vi "PID Calculate Gains.vi"(3 "PID parameters":cluster{"Kc":dbl, "Ti":dbl, "Td":dbl} {"Td" format="%.2f"; "Ti" format="%.2f"; "Kc" format="%.2f"}, 4 "autotuning parameters":T1={"Controller Type"=0, "# of cycles to avg"=3, "Relay amplitude (%)"=0.0, "Control design  "=0, "Noise level %"=0.25} {"Noise level %" format="%.2f"; "Control design" items=["Normal", "Fast", "Slow"]; "Relay amplitude (%)" format="%.2f"; "Controller Type" items=["PID", "PI", "P"]}, 5 "Mean amplitude":dbl format="%.2f", 6 "Mean period":dbl format="%.2f") -> (0 "tuned PID parameters":cluster{"Kc":dbl, "Ti":dbl, "Td":dbl} {"Td" format="%.2f"; "Ti" format="%.2f"; "Kc" format="%.2f"}, 1 "Tu":dbl format="%.2f", 2 "Kr":dbl)   [LabVIEW 2020, in "NI_PID_autopid.lvlib"]
doc: "This VI determines the new PID parameters from the results of the setpoint relay experiment."
uses:
  <vilib>/addons/control/pid/NI_PID_autopid.lvlib
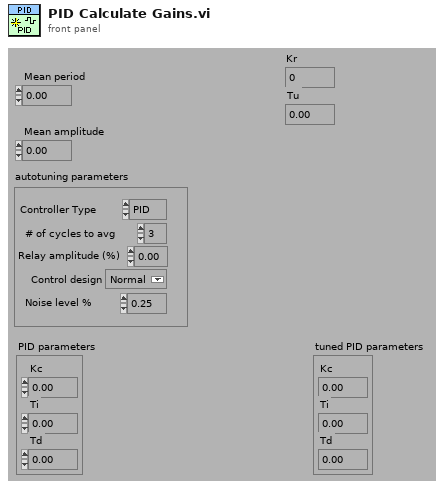
[diagram p1: front panel]
types:
  T1 = cluster{"Controller Type":u16, "# of cycles to avg":i32, "Relay amplitude (%)":dbl, "Control design  ":u16, "Noise level %":dbl}
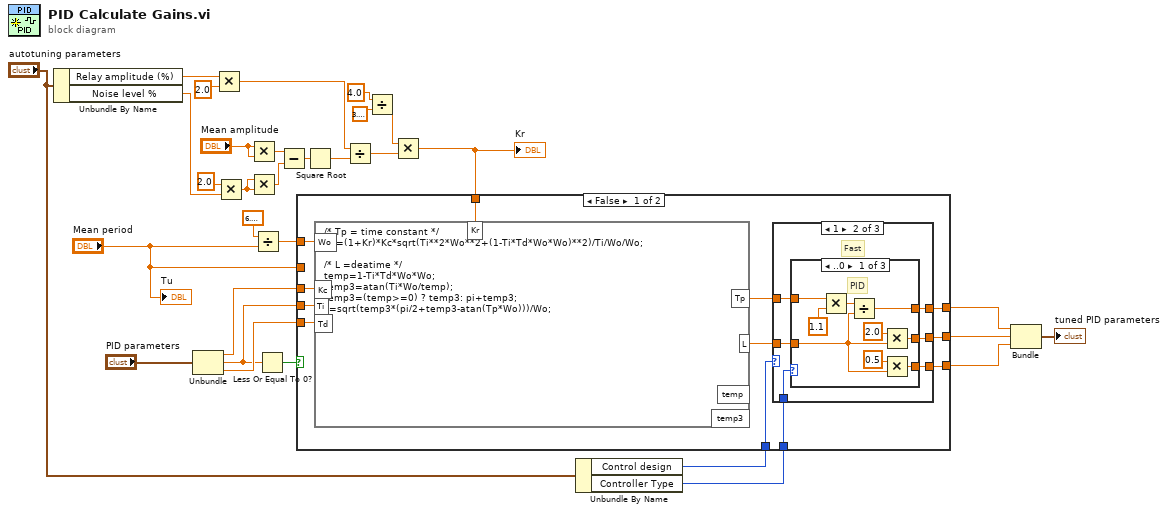
[diagram p0: block diagram]
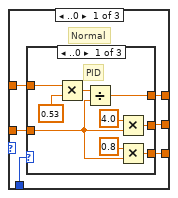
[diagram p2: hidden frame]
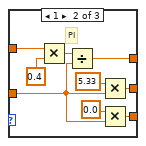
[diagram p3: hidden frame]
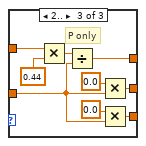
[diagram p4: hidden frame]
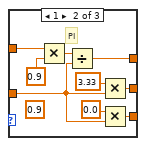
[diagram p5: hidden frame]
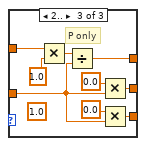
[diagram p6: hidden frame]
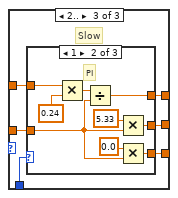
[diagram p7: hidden frame]
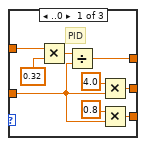
[diagram p8: hidden frame]
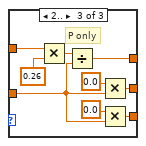
[diagram p9: hidden frame]
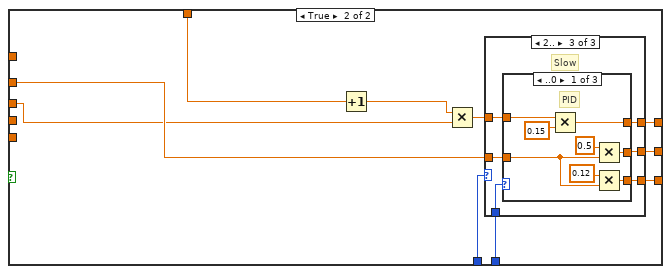
[diagram p10: hidden frame]
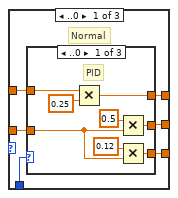
[diagram p11: hidden frame]
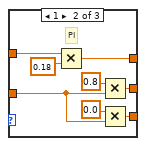
[diagram p12: hidden frame]
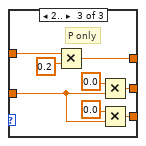
[diagram p13: hidden frame]
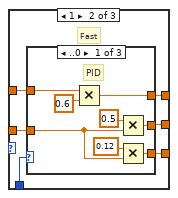
[diagram p14: hidden frame]
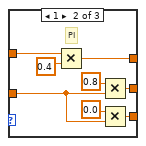
[diagram p15: hidden frame]
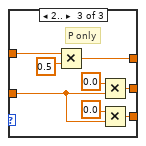
[diagram p16: hidden frame]
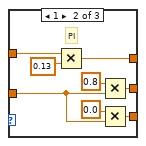
[diagram p17: hidden frame]
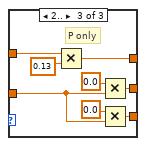
[diagram p18: hidden frame]
diagram:
  n1 = Unbundle By Name("autotuning parameters") -> ("Relay amplitude (%)"=w15:dbl, "Noise level %"=w1:dbl)
  n2 = Unbundle("PID parameters") -> ("Kc"=w5:dbl, "Ti"=w19:dbl, "Td"=w20:dbl)
  n3 = Multiply(x=w15, y=2.0) -> (x*y=w29:dbl)
  n4 = Multiply(x=2.0, y=w1) -> (x*y=w24:dbl)
  n5 = Multiply(x="Mean amplitude", y="Mean amplitude") -> (x*y=w26:dbl)
  n6 = Multiply(x=w24, y=w24) -> (x*y=w22:dbl)
  n7 = Divide(x=6.283185307179586, y="Mean period") -> (x/y=w8:dbl)
  n8 = Less Or Equal To 0?(x=w19) -> (x <= 0?=w30:bool)
  n9 = Subtract(x=w26, y=w22) -> (x-y=w23:dbl)
  n10 = Square Root(x=w23) -> (sqrt(x)=w25:dbl)
  n11 = Divide(x=w29, y=w25) -> (x/y=w27:dbl)
  n12 = Divide(x=4.0, y=3.141592653589793) -> (x/y=w11:dbl)
  n13 = Multiply(x=w11, y=w27) -> (x*y=w28:dbl)
  "Kr" <- w28
  n14 = Unbundle By Name("autotuning parameters") -> ("Control design"=w10:u16, "Controller Type"=w9:u16)
  n15 = case shown="False" w30 {
    tunnel: w20 -> [w43 _]
    tunnel: w19 -> [w42 _]
    tunnel: w28 -> [w41 w148]
    tunnel: [w34 w146] -> w4
    tunnel: [w33 w145] -> w21
    tunnel: w5 -> [w40 w143]
    tunnel: w10 -> [w37 w152]
    tunnel: w9 -> [w36 w151]
    tunnel: w8 -> [w35 _]
    tunnel: "Mean period" -> [_ w150]
    tunnel: [w32 w144] -> w6
    frame False {
      n16 = formula code="/* Tp = time constant */\nTp=(1+Kr)*Kc*sqrt(Ti**2*Wo**2+(1-Ti*Td*Wo*Wo)**2)/Ti/Wo/Wo;\n\n/* L =deatime */\ntemp=1-Ti*Td*Wo*Wo;\ntemp3=atan(Ti*Wo/temp);\ntemp3=(temp>=0) ? temp3: pi+temp3;\nL=sqrt(temp3*(pi/2+temp3-atan(Tp*Wo)))/Wo;"("Wo"=w35, "Kr"=w41, "Ti"=w42, "Td"=w43, "Kc"=w40) -> ("Tp"=w38:dbl, "L"=w39:dbl)  [unwired: 2 out]
      n17 = case shown="1" w37 {
        tunnel: [w49 w78 w113] -> w33
        tunnel: [w48 w79 w114] -> w32
        tunnel: [w47 w80 w115] -> w34
        tunnel: w39 -> [w46 w81 w112]
        tunnel: w38 -> [w45 w82 w111]
        tunnel: w36 -> [w44 w77 w110]
        frame ..0 {
          # "Normal"
          n18 = case shown="..0" w44 {
            tunnel: [w50 w59 w68] -> w47
            tunnel: [w55 w64 w73] -> w49
            tunnel: w46 -> [w54 w63 w72]
            tunnel: [w51 w60 w69] -> w48
            tunnel: w45 -> [w52 w61 w70]
            frame ..0 {
              # "PID"
              n19 = Multiply(x=w52, y=0.53) -> (x*y=w58:dbl)
              n20 = Divide(x=w58, y=w54) -> (x/y=w50:dbl)
              n21 = Multiply(x=4.0, y=w54) -> (x*y=w51:dbl)
              n22 = Multiply(x=0.8, y=w54) -> (x*y=w55:dbl)
            }
            frame 1 {
              # "PI"
              n23 = Multiply(x=w61, y=0.4) -> (x*y=w67:dbl)
              n24 = Divide(x=w67, y=w63) -> (x/y=w59:dbl)
              n25 = Multiply(x=5.33, y=w63) -> (x*y=w60:dbl)
              n26 = Multiply(x=0.0, y=w63) -> (x*y=w64:dbl)
            }
            frame 2.. {
              # "P only"
              n27 = Multiply(x=w70, y=0.44) -> (x*y=w76:dbl)
              n28 = Divide(x=w76, y=w72) -> (x/y=w68:dbl)
              n29 = Multiply(x=0.0, y=w72) -> (x*y=w69:dbl)
              n30 = Multiply(x=0.0, y=w72) -> (x*y=w73:dbl)
            }
          }
        }
        frame 1 {
          # "Fast"
          n31 = case shown="..0" w77 {
            tunnel: [w83 w92 w101] -> w80
            tunnel: [w88 w97 w106] -> w78
            tunnel: w81 -> [w87 w96 w105]
            tunnel: [w84 w93 w102] -> w79
            tunnel: w82 -> [w85 w94 w103]
            frame ..0 {
              # "PID"
              n32 = Multiply(x=w85, y=1.1) -> (x*y=w91:dbl)
              n33 = Divide(x=w91, y=w87) -> (x/y=w83:dbl)
              n34 = Multiply(x=2.0, y=w87) -> (x*y=w84:dbl)
              n35 = Multiply(x=0.5, y=w87) -> (x*y=w88:dbl)
            }
            frame 1 {
              (unwired) 0.9
              # "PI"
              n36 = Multiply(x=w94, y=0.9) -> (x*y=w100:dbl)
              n37 = Divide(x=w100, y=w96) -> (x/y=w92:dbl)
              n38 = Multiply(x=3.33, y=w96) -> (x*y=w93:dbl)
              n39 = Multiply(x=0.0, y=w96) -> (x*y=w97:dbl)
            }
            frame 2.. {
              (unwired) 1.0
              # "P only"
              n40 = Multiply(x=w103, y=1.0) -> (x*y=w109:dbl)
              n41 = Divide(x=w109, y=w105) -> (x/y=w101:dbl)
              n42 = Multiply(x=0.0, y=w105) -> (x*y=w102:dbl)
              n43 = Multiply(x=0.0, y=w105) -> (x*y=w106:dbl)
            }
          }
        }
        frame 2.. {
          # "Slow"
          n44 = case shown="1" w110 {
            tunnel: [w116 w125 w134] -> w115
            tunnel: [w121 w130 w139] -> w113
            tunnel: w112 -> [w120 w129 w138]
            tunnel: [w117 w126 w135] -> w114
            tunnel: w111 -> [w118 w127 w136]
            frame ..0 {
              # "PID"
              n45 = Multiply(x=w118, y=0.32) -> (x*y=w124:dbl)
              n46 = Divide(x=w124, y=w120) -> (x/y=w116:dbl)
              n47 = Multiply(x=4.0, y=w120) -> (x*y=w117:dbl)
              n48 = Multiply(x=0.8, y=w120) -> (x*y=w121:dbl)
            }
            frame 1 {
              # "PI"
              n49 = Multiply(x=w127, y=0.24) -> (x*y=w133:dbl)
              n50 = Divide(x=w133, y=w129) -> (x/y=w125:dbl)
              n51 = Multiply(x=5.33, y=w129) -> (x*y=w126:dbl)
              n52 = Multiply(x=0.0, y=w129) -> (x*y=w130:dbl)
            }
            frame 2.. {
              # "P only"
              n53 = Multiply(x=w136, y=0.26) -> (x*y=w142:dbl)
              n54 = Divide(x=w142, y=w138) -> (x/y=w134:dbl)
              n55 = Multiply(x=0.0, y=w138) -> (x*y=w135:dbl)
              n56 = Multiply(x=0.0, y=w138) -> (x*y=w139:dbl)
            }
          }
        }
      }
    }
    frame True {
      n57 = Increment(x=w148) -> (x+1=w147:dbl)
      n58 = Multiply(x=w147, y=w143) -> (x*y=w149:dbl)
      n59 = case shown="2.." w152 {
        tunnel: [w158 w188 w218] -> w145
        tunnel: [w157 w187 w217] -> w144
        tunnel: [w156 w186 w216] -> w146
        tunnel: w150 -> [w155 w185 w215]
        tunnel: w149 -> [w154 w184 w214]
        tunnel: w151 -> [w153 w183 w213]
        frame ..0 {
          # "Normal"
          n60 = case shown="..0" w153 {
            tunnel: [w159 w167 w175] -> w156
            tunnel: [w164 w172 w180] -> w158
            tunnel: w155 -> [w163 w171 w179]
            tunnel: [w160 w168 w176] -> w157
            tunnel: w154 -> [w161 w169 w177]
            frame ..0 {
              # "PID"
              n61 = Multiply(x=w161, y=0.25) -> (x*y=w159:dbl)
              n62 = Multiply(x=0.5, y=w163) -> (x*y=w160:dbl)
              n63 = Multiply(x=0.12, y=w163) -> (x*y=w164:dbl)
            }
            frame 1 {
              # "PI"
              n64 = Multiply(x=w169, y=0.18) -> (x*y=w167:dbl)
              n65 = Multiply(x=0.8, y=w171) -> (x*y=w168:dbl)
              n66 = Multiply(x=0.0, y=w171) -> (x*y=w172:dbl)
            }
            frame 2.. {
              # "P only"
              n67 = Multiply(x=w177, y=0.2) -> (x*y=w175:dbl)
              n68 = Multiply(x=0.0, y=w179) -> (x*y=w176:dbl)
              n69 = Multiply(x=0.0, y=w179) -> (x*y=w180:dbl)
            }
          }
        }
        frame 1 {
          # "Fast"
          n70 = case shown="..0" w183 {
            tunnel: [w189 w197 w205] -> w186
            tunnel: [w194 w202 w210] -> w188
            tunnel: w185 -> [w193 w201 w209]
            tunnel: [w190 w198 w206] -> w187
            tunnel: w184 -> [w191 w199 w207]
            frame ..0 {
              # "PID"
              n71 = Multiply(x=w191, y=0.6) -> (x*y=w189:dbl)
              n72 = Multiply(x=0.5, y=w193) -> (x*y=w190:dbl)
              n73 = Multiply(x=0.12, y=w193) -> (x*y=w194:dbl)
            }
            frame 1 {
              # "PI"
              n74 = Multiply(x=w199, y=0.4) -> (x*y=w197:dbl)
              n75 = Multiply(x=0.8, y=w201) -> (x*y=w198:dbl)
              n76 = Multiply(x=0.0, y=w201) -> (x*y=w202:dbl)
            }
            frame 2.. {
              # "P only"
              n77 = Multiply(x=w207, y=0.5) -> (x*y=w205:dbl)
              n78 = Multiply(x=0.0, y=w209) -> (x*y=w206:dbl)
              n79 = Multiply(x=0.0, y=w209) -> (x*y=w210:dbl)
            }
          }
        }
        frame 2.. {
          # "Slow"
          n80 = case shown="..0" w213 {
            tunnel: [w219 w227 w235] -> w216
            tunnel: [w224 w232 w240] -> w218
            tunnel: w215 -> [w223 w231 w239]
            tunnel: [w220 w228 w236] -> w217
            tunnel: w214 -> [w221 w229 w237]
            frame ..0 {
              # "PID"
              n81 = Multiply(x=w221, y=0.15) -> (x*y=w219:dbl)
              n82 = Multiply(x=0.5, y=w223) -> (x*y=w220:dbl)
              n83 = Multiply(x=0.12, y=w223) -> (x*y=w224:dbl)
            }
            frame 1 {
              # "PI"
              n84 = Multiply(x=w229, y=0.13) -> (x*y=w227:dbl)
              n85 = Multiply(x=0.8, y=w231) -> (x*y=w228:dbl)
              n86 = Multiply(x=0.0, y=w231) -> (x*y=w232:dbl)
            }
            frame 2.. {
              # "P only"
              n87 = Multiply(x=w237, y=0.13) -> (x*y=w235:dbl)
              n88 = Multiply(x=0.0, y=w239) -> (x*y=w236:dbl)
              n89 = Multiply(x=0.0, y=w239) -> (x*y=w240:dbl)
            }
          }
        }
      }
    }
  }
  n90 = Bundle(w4, w6, w21) -> (→"tuned PID parameters":cluster{dbl, dbl, dbl})  [unwired: 1 out]
  "Tu" <- "Mean period"
